vi "FGV.vi"(0 "Simulada in":refnum<class "Simulada.lvclass">, 1 "Enum":enum16{"Get Data", "Set Data"}(ring), 2 "Name":string, 3 "error in (no error)":errorcluster, 4 "Data 2":variant) -> (7 "Simulada out":refnum<class "Simulada.lvclass">, 9 "Data":variant, 10 "error out":errorcluster)   [LabVIEW 2020, in "Simulada.lvclass"]
uses:
  Simulada.lvclass
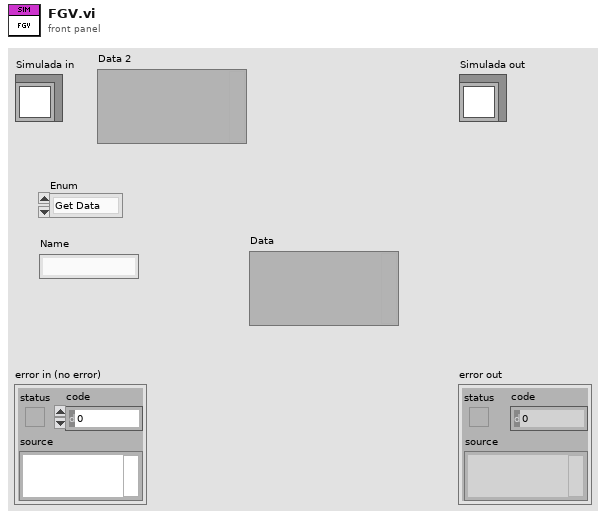
[diagram p1: front panel]
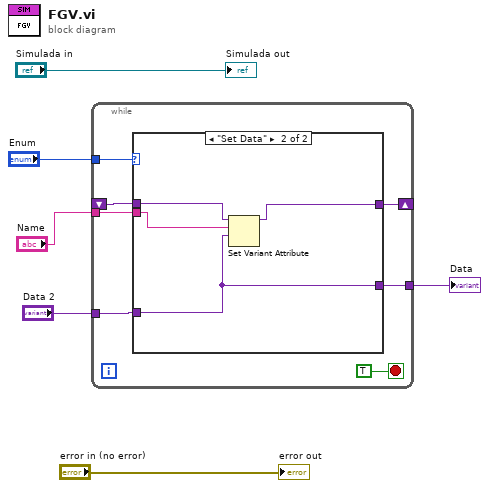
[diagram p0: block diagram]
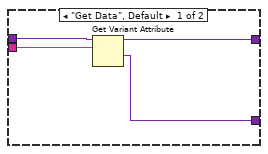
[diagram p2: hidden frame]
diagram:
  n1 = while {
    tunnel: "Enum" -> [w12]
    tunnel: "Name" -> [w11]
    tunnel: "Data 2" -> [w10]
    shift-right: [w9] -> _
    shift-left: _ -> [w8]
    tunnel: [w7] -> w1
    stop <- TRUE stop-if-true
    n2 = case shown="\"Set Data\"" w12 {
      tunnel: w11 -> [w17 w20]
      tunnel: w10 -> [_ w18]
      tunnel: [w16 w19] -> w9
      tunnel: w8 -> [w15 w21]
      tunnel: [w14 w18] -> w7
      frame "Get Data", Default {
        n3 = Get Variant Attribute(Variant=w15, name=w17) -> (duplicate Variant=w16:variant, value=w14:variant)  [unwired: 2 in, 2 out]
      }
      frame "Set Data" {
        n4 = Set Variant Attribute(Variant=w21, name=w20, value=w18) -> (Variant out=w19:variant)  [unwired: 1 in, 2 out]
      }
    }
  }
  "Data" <- w1
  "error out" <- "error in (no error)"
  "Simulada out" <- "Simulada in"
